vi "Q - even.vi"(11 "Numeric":i32) -> (2 "even ?":bool, 3 "saw":i32)   [LabVIEW 2015]
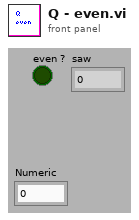
[diagram p1: front panel]
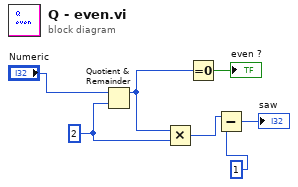
[diagram p0: block diagram]
diagram:
  w4 = 2 ("y")
  n1 = Quotient & Remainder(x="Numeric", y=w4) -> (x-y*floor(x/y)=w5:i32)  [unwired: 1 out]
  n2 = Multiply(x=w5, y=w4) -> (x*y=w3:i32)
  n3 = Equal To 0?(x=w5) -> (x = 0?=→"even ?":bool)
  n4 = Subtract(x=w3, y=1) -> (x-y=→"saw":i32)
